vi "Example Main Program.vi"() -> ()   [LabVIEW 2018]
uses:
  Example Logging Cluster.ctl
  Example Logging Data.ctl
  File Headers Array.ctl
  Target Metadata Headers Array.ctl
  Target Timing and Logging Init Cluster.ctl
  <vilib>/ptbypt/NI_PtbyPt.lvlib
  COBRA Logging and Loop Timing Library.lvlib
panel:
  out "Target Data Logging Active":bool
  in  "Start Log":bool
  in  "File Name":string
  out "Waveform Chart":cluster{"Sine":dbl, "Cosine":dbl}(graph)={"Sine"=1.9960534568565433, "Cosine"=0.12558103905862825}
  in  "Stop":bool
  in  "Sine Wave Params":cluster{"Amplitude":dbl, "Frequency (Hz)":dbl}={"Amplitude"=2.0, "Frequency (Hz)"=1.0}
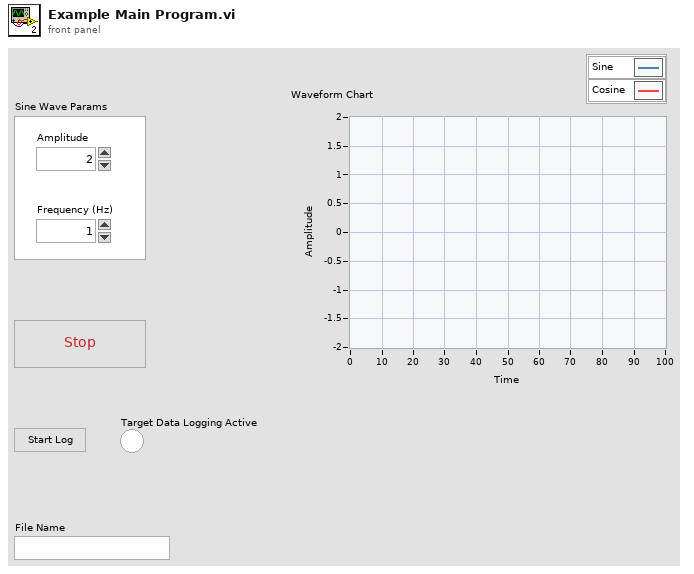
[diagram p1: front panel]
types:
  T1 = typedef "COBRA Logging and Loop Timing Library.lvlib/Target Metadata Headers Array.ctl" = string[]
  T2 = typedef "COBRA Logging and Loop Timing Library.lvlib/File Headers Array.ctl" = string[]
  T3 = typedef "COBRA Logging and Loop Timing Library.lvlib/Target Timing and Logging Init Cluster.ctl" = cluster{"Target Period (uS)":dbl, "Target Logging Duration (s)":dbl, "Target File Path":string, "Target File Headers":T2, "Target Metadata File Headers":T1}
  T4 = typedef "Example Logging Cluster.ctl" = cluster{"Valid for Logging?":bool, "Logging Data":T5}
  T5 = typedef "Example Logging Data.ctl" = cluster{"Sine":dbl, "Cosine":dbl}
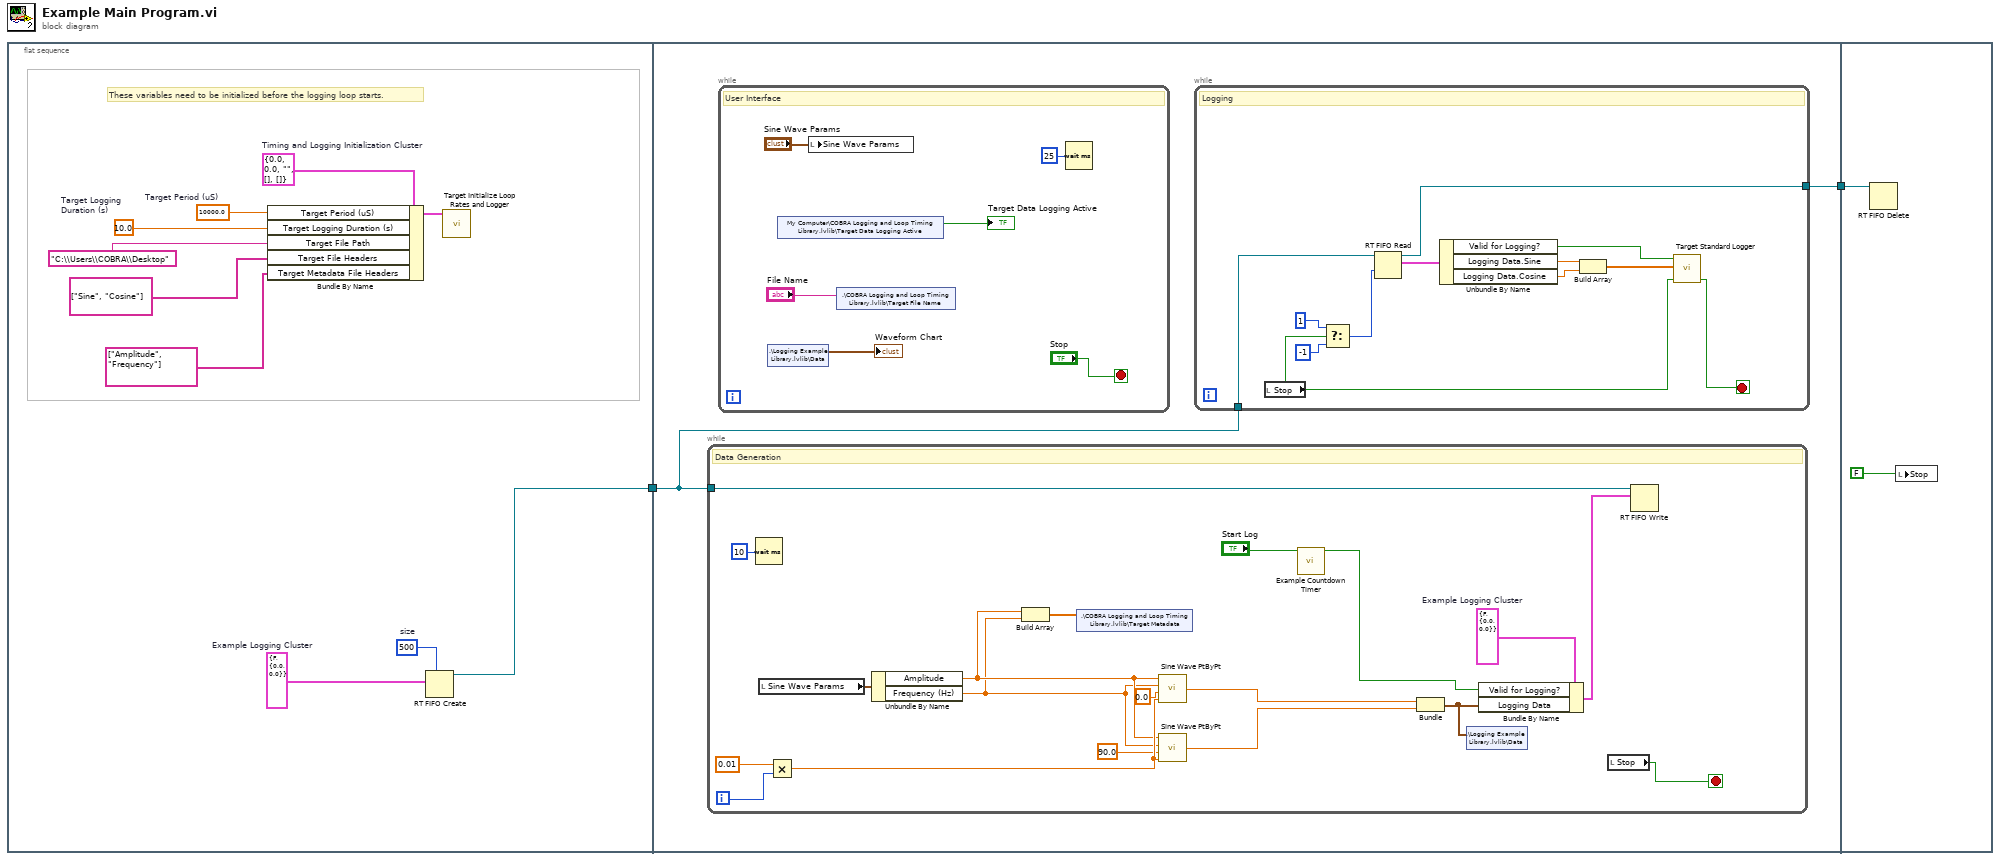
[diagram p0: block diagram]
diagram:
  n1 = flat-sequence {
    tunnel: [w10] -> w2
    tunnel: w2 -> [w14]
    tunnel: [w13] -> w1
    tunnel: w1 -> [w52]
    frame #0 {
      w9 = T3 {"Target Period (uS)"=0.0, "Target Logging Duration (s)"=0.0, "Target File Path"="", "Target File Headers"=[], "Target Metadata File Headers"=[]}  # Timing and Logging Initialization Cluster
      w7 = 10000.0  # Target Period (uS)
      w6 = 10.0  # Target Logging Duration (s)
      w11 = u32 500  # size
      w12 = T4 {"Valid for Logging?"=FALSE, "Logging Data"={"Sine"=0.0, "Cosine"=0.0}}  # Example Logging Cluster
      # "These variables need to be initialized before the logging loop starts."
      n2 = Bundle By Name(cluster=w9, "Target Period (uS)"=w7, "Target Logging Duration (s)"=w6, "Target File Path"="C:\\Users\\COBRA\\Desktop", "Target File Headers"=T2 ["Sine", "Cosine"], "Target Metadata File Headers"=T1 ["Amplitude", "Frequency"]) -> (w8:T3)
      n3 = RT FIFO Create(1:w12, 4:w11) -> (8:w10:refnum<k33>)  [unwired: 6 in, 2 out]
      n4 = call "Target Initialize Loop Rates and Logger.vi"("Timing and Logging Initialization Cluster"=w8) -> ()  [unwired: 11 in]
    }
    frame #1 {
      n5 = while {
        tunnel: w14 -> [w42]
        i -> [w49]
        stop <- w40 stop-if-true
        w45 = T4 {"Valid for Logging?"=FALSE, "Logging Data"={"Sine"=0.0, "Cosine"=0.0}}  # Example Logging Cluster
        # "Data Generation"
        n6 = Wait (ms)(milliseconds to wait=u32 10) -> ()  [unwired: 1 out]
        n7 = local read "Sine Wave Params"() -> (w48:cluster{"Amplitude":dbl, "Frequency (Hz)":dbl})
        n8 = Multiply(x=0.01, y=w49) -> (x*y=w47:dbl)
        n9 = Unbundle By Name(w48) -> ("Amplitude"=w38:dbl, "Frequency (Hz)"=w37:dbl)
        n10 = Build Array(w38, w37) -> (w36:dbl[])
        n11 = shared-variable ".\\COBRA Logging and Loop Timing Library.lvlib\\Target Metadata"(w36) -> ()  [unwired: 1 in, 1 out]
        n12 = call <vilib>:"Sine Wave PtByPt.vi"("time"=w47, "phase"=0.0, "frequency"=w37, "amplitude"=w38) -> ("sine wave"=w44:dbl)
        n13 = call <vilib>:"Sine Wave PtByPt.vi"("time"=w47, "phase"=90.0, "frequency"=w37, "amplitude"=w38) -> ("sine wave"=w43:dbl)
        n14 = call "Example Countdown Timer.vi"("Start Logging"="Start Log") -> ("Valid for Logging"=w33:bool)  [unwired: 10 in]
        n15 = Bundle("sine wave"=w44, "sine wave"=w43) -> (w39:cluster{"sine wave":dbl, "sine wave":dbl})  [unwired: 1 in]
        n16 = shared-variable ".\\Logging Example Library.lvlib\\Data"(w39) -> ()  [unwired: 1 in, 1 out]
        n17 = Bundle By Name(cluster=w45, "Valid for Logging?"=w33, "Logging Data"=w39) -> (w41:T4)
        n18 = local read "Stop"() -> (w40:bool)
        n19 = RT FIFO Write(0:w42, 1:w41) -> ()  [unwired: 3 in, 4 out]
      }
      n20 = while {
        stop <- "Stop" stop-if-true
        # "User Interface"
        n21 = shared-variable ".\\Logging Example Library.lvlib\\Data"() -> (→"Waveform Chart":T5)  [unwired: 1 in, 1 out]
        n22 = shared-variable "My Computer\\COBRA Logging and Loop Timing Library.lvlib\\Target Data Logging Active"() -> (→"Target Data Logging Active":bool)  [unwired: 1 in, 1 out]
        n23 = local write "Sine Wave Params"("Sine Wave Params") -> ()
        n24 = shared-variable ".\\COBRA Logging and Loop Timing Library.lvlib\\Target File Name"("File Name") -> ()  [unwired: 1 in, 1 out]
        n25 = Wait (ms)(milliseconds to wait=u32 25) -> ()  [unwired: 1 out]
      }
      n26 = while {
        tunnel: w14 -> [w32]
        tunnel: [w21] -> w13
        stop <- w22 stop-if-true
        # "Logging"
        n27 = local read "Stop"() -> (w23:bool)
        n28 = Select(t=1, s=w23, f=-1) -> (s? t:f=w24:i32)
        n29 = RT FIFO Read(0:w32, 2:w24) -> (8:w21:refnum<k33>, 9:w31:T4)  [unwired: 2 in, 3 out]
        n30 = Unbundle By Name(w31) -> ("Valid for Logging?"=w27:bool, "Logging Data.Sine"=w30:dbl, "Logging Data.Cosine"=w29:dbl)
        n31 = Build Array(w30, w29) -> (w28:dbl[])
        n32 = call "Target Standard Logger.vi"("Stop Command"=w23, "Incoming Data Array"=w28, "Valid for Logging?"=w27) -> ("Ok to Stop Logging Loop"=w22:bool)  [unwired: 8 in]
      }
    }
    frame #2 {
      n33 = RT FIFO Delete(0:w52) -> ()  [unwired: 2 in, 1 out]
      n34 = local write "Stop"(FALSE ("Stop")) -> ()
    }
  }
